vi "OpenCVCam_ClassCast.vi"(11 "OpenCVCamIn":refnum<class>) -> (3 "OpenCVCamOut":refnum<class "OpenCVCam.lvclass">)   [LabVIEW 2021, in "OpenCVCam.lvclass"]
uses:
  OpenCVCam.lvclass
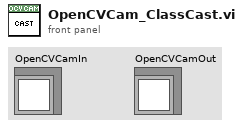
[diagram p1: front panel]
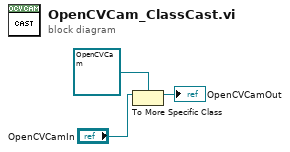
[diagram p0: block diagram]
diagram:
  n1 = To More Specific Class(target class=refnum<class "OpenCVCam.lvclass"> refnum ("reference in"), reference="OpenCVCamIn") -> (specific class reference=→"OpenCVCamOut":refnum<class "OpenCVCam.lvclass">)  [unwired: 1 in, 1 out]
